vi "Draw.vi"(8 "error in (no error)":errorcluster, 10 "RT_Game.lvlib:Game.lvclass":refnum<class "Game.lvclass">, 11 "BounceTarget in":refnum<class "BounceTarget.lvclass">) -> (0 "error out":errorcluster, 2 "RT_Game.lvlib:Game.lvclass 2":refnum<class "Game.lvclass">, 3 "BounceTarget out":refnum<class "BounceTarget.lvclass">)   [LabVIEW 2019, in "RT_Game.lvlib" / "BounceTarget.lvclass"]
uses:
  BounceTarget.lvclass
  C:/Users/FreshBob/Dropbox/VIs/myRIO_GameConsole/RT/RT_Game/GameObject/GameObject.lvclass
  Game/Game.lvclass
  BounceTarget.lvclass/BounceTarget.ctl
  GameObject/GameObject.lvclass/GameObject.ctl
  GameObject/Read size.vi
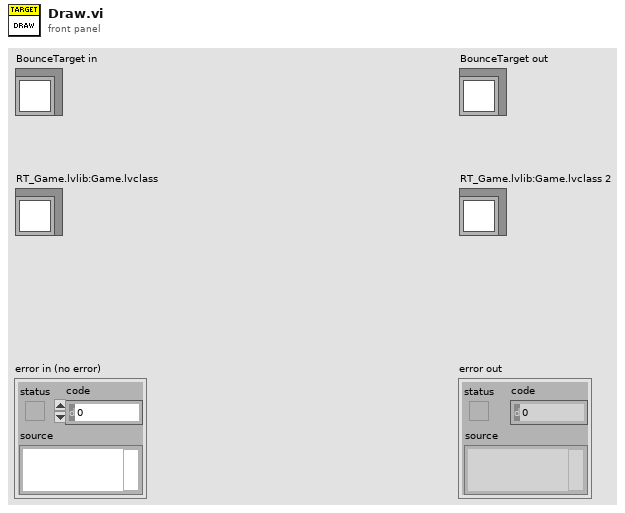
[diagram p1: front panel]
types:
  T1 = typedef "RT_Game.lvlib/Game.lvclass/Coordinate.ctl" = cluster{"x":dbl, "y":dbl}
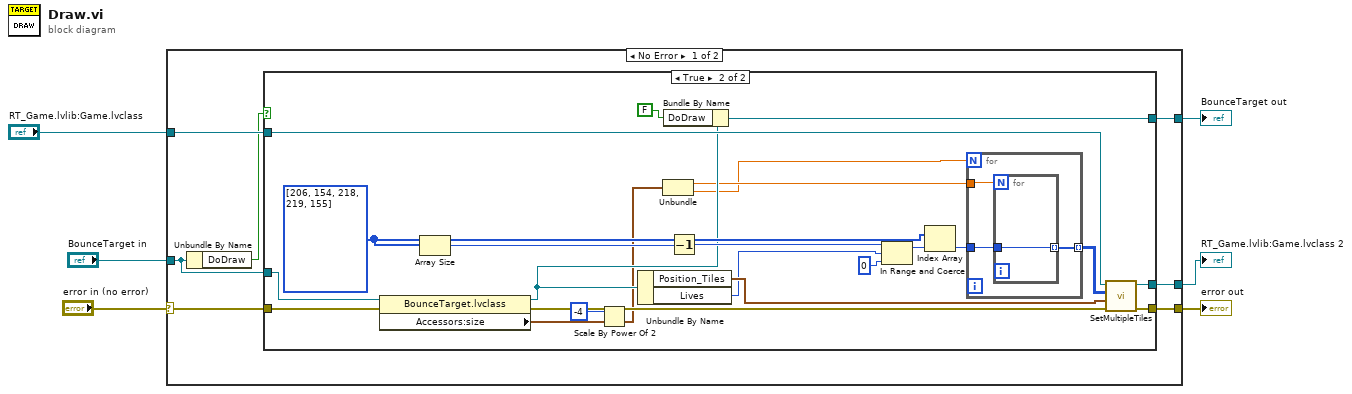
[diagram p0: block diagram]
diagram:
  n1 = case shown="No Error" "error in (no error)" {
    selector: "error in (no error)" -> [w13 w46]
    tunnel: [w12 w46] -> w5
    tunnel: [w7 w45] -> w3
    tunnel: "BounceTarget in" -> [w9 w45]
    tunnel: [w11 w44] -> w1
    tunnel: "RT_Game.lvlib:Game.lvclass" -> [w10 w44]
    frame No Error {
      n2 = Unbundle By Name(w9) -> ("DoDraw"=w8:bool)
      n3 = case shown="True" w8 {
        tunnel: w13 -> [w15 w39]
        tunnel: [w15 w38] -> w12
        tunnel: [w16 w37] -> w11
        tunnel: w10 -> [w16 w36]
        tunnel: w9 -> [w14 w28]
        tunnel: [w14 w31] -> w7
        frame False {
        }
        frame True {
          w34 = u32[] [206, 154, 218, 219, 155] ("replace_color")
          n4 = property class="BounceTarget.lvclass"(reference=w28, error in=w39) -> (reference out=w27:refnum<class "BounceTarget.lvclass">, error out=w29:errorcluster, "Accessors:size"=w26:T1)
          n5 = Array Size(array=w34) -> (size(s)=w33:i32)
          n6 = Scale By Power Of 2(n=i16 -4, x=w26) -> (x*2^n=w23:T1)
          n7 = Unbundle By Name(w27) -> ("Position_Tiles"=w35:T1, "Lives"=w21:i16)
          n8 = Unbundle(w23) -> ("x"=w25:dbl, "y"=w24:dbl)
          n9 = Bundle By Name(cluster=w27, "DoDraw"=FALSE) -> (w31:refnum<class "BounceTarget.lvclass">)
          n10 = Decrement(x=w33) -> (x-1=w32:i32)
          n11 = In Range and Coerce(upper limit=w32, x=w21, lower limit=i16 0) -> (coerced(x)=w18:i32)  [unwired: 1 out]
          n12 = Index Array(array=w34, index=w18) -> (element=w19:u32)
          n13 = for {
            N: w24 -> [_]
            tunnel: w19 -> [w42]
            tunnel: [w41] -> w20 mode=indexing
            tunnel: w25 -> [w40]
            n14 = for {
              N: w40 -> [_]
              tunnel: w42 -> [w43]
              tunnel: [w43] -> w41 mode=indexing
            }
          }
          n15 = call "SetMultipleTiles.vi"("error in (no error)"=w29, "Position"=w35, "TileCodes"=w20, "Game in"=w36) -> ("error out"=w38:errorcluster, "Game out"=w37:refnum<class "Game.lvclass">)  [unwired: 6 in]
        }
      }
    }
    frame Error {
    }
  }
  "error out" <- w5
  "BounceTarget out" <- w3
  "RT_Game.lvlib:Game.lvclass 2" <- w1
